vi "Set Friction.vi"(7 "Viscous Friction":dbl, 8 "error in (no error)":errorcluster, 9 "Negative Coulomb Friction":dbl, 10 "Positive Coulomb Friction":dbl, 11 "Link in":refnum<class "Link.lvclass">) -> (0 "error out":errorcluster, 3 "Link out":refnum<class "Link.lvclass">)   [LabVIEW 2013, in "Link.lvclass"]
uses:
  Link.lvclass
  Link.lvclass/Link.ctl
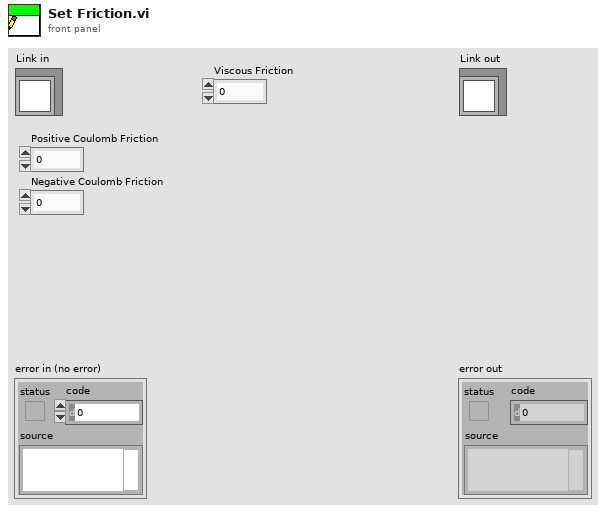
[diagram p1: front panel]
types:
  T1 = cluster{"Positive Coulomb Friction":dbl, "Negative Coulomb Friction":dbl}
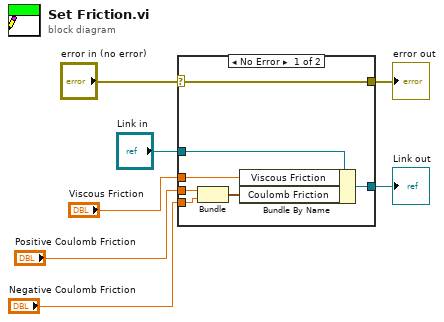
[diagram p0: block diagram]
diagram:
  n1 = case shown="No Error" "error in (no error)" {
    selector: "error in (no error)" -> [w14 w15]
    tunnel: [w14 w15] -> w6
    tunnel: [w12 w16] -> w4
    tunnel: "Link in" -> [w13 w16]
    tunnel: "Negative Coulomb Friction" -> [w10 _]
    tunnel: "Positive Coulomb Friction" -> [w9 _]
    tunnel: "Viscous Friction" -> [w8 _]
    frame No Error {
      n2 = Bundle("Positive Coulomb Friction"=w9, "Negative Coulomb Friction"=w10) -> (w11:T1)  [unwired: 1 in]
      n3 = Bundle By Name(cluster=w13, "Viscous Friction"=w8, "Coulomb Friction"=w11) -> (w12:refnum<class "Link.lvclass">)
    }
    frame Error {
    }
  }
  "error out" <- w6
  "Link out" <- w4
